vi "Setup.vi"(0 "Vector Path in":refnum<class "Vector 18GHz Path.lvclass">, 11 "error in":errorcluster) -> (4 "Vector Path out":refnum<class "Vector 18GHz Path.lvclass">, 15 "error out":errorcluster)   [LabVIEW 2023, in "RFFixtureCharact.RFPM.lvlib" / "Vector 18GHz Path.lvclass"]
uses:
  Vector 18GHz Path.lvclass
  C:/rfcal/AuxTools/STSRFFixtureCharactUtility/Source/Code Modules/Common/Base Classes/Path/Path.lvclass
  Public/Base Classes/Vector/Vector Abstract Path/Vector Abstract Path.lvclass
  Vector 18GHz Path.lvclass/Vector 18GHz Path.ctl
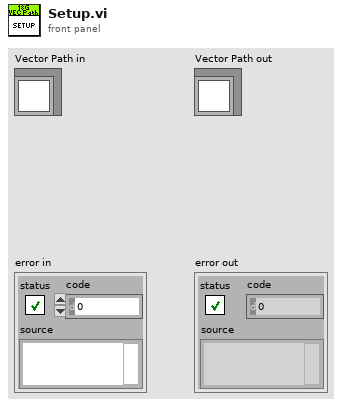
[diagram p1: front panel]
types:
  T1 = typedef "RFFixtureCharact.RFPM.lvlib/Vector 18GHz Path Group.lvclass/Sweep.ctl" = cluster{"Port Power":dbl, "Frequencies":dbl[], "Reference Level":dbl, "IF Bandwidth":dbl}
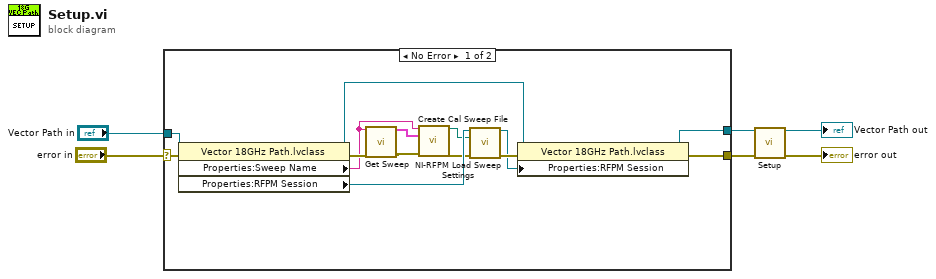
[diagram p0: block diagram]
diagram:
  n1 = case shown="No Error" "error in" {
    selector: "error in" -> [w20 w22]
    tunnel: [w16 w22] -> w1
    tunnel: [w17 w21] -> w2
    tunnel: "Vector Path in" -> [w15 w21]
    frame No Error {
      n2 = property class="Vector 18GHz Path.lvclass"(reference=w15, error in=w20) -> (reference out=w18:refnum<class "Vector 18GHz Path.lvclass">, error out=w11:errorcluster, "Properties:Sweep Name"=w7:string, "Properties:RFPM Session"=w14:refnum<k15>)
      n3 = call "Get Sweep.vi"("Sweep Name"=w7, "error in (no error)"=w11) -> ("Grid"=w8:T1, "error out"=w12:errorcluster)  [unwired: 11 in, 1 out]
      n4 = call "Create Cal Sweep File.vi"("Sweep Name"=w7, "Grid"=w8, "error in (no error)"=w12) -> ("Sweep File Path"=w9:path, "error out"=w10:errorcluster)  [unwired: 11 in]
      n5 = call <instrlib>:"NI-RFPM Load Sweep Settings.vi"("instrument handle"=w14, "Sweep Settings File Path"=w9, "error in"=w10) -> ("instrument handle out"=w13:refnum<k15>, "error out"=w19:errorcluster)  [unwired: 11 in]
      n6 = property class="Vector 18GHz Path.lvclass"(reference=w18, error in=w19, "Properties:RFPM Session"=w13) -> (reference out=w17:refnum<class "Vector 18GHz Path.lvclass">, error out=w16:errorcluster)
    }
    frame Error {
    }
  }
  n7 = call-parent "Setup.vi"("Vector Path in"=w2, "error in (no error)"=w1) -> ("Vector Path out"=→"Vector Path out":refnum<class "Vector 18GHz Path.lvclass">, "error out"=→"error out":errorcluster)  [unwired: 12 in]
